vi "main_ctrl.vi"(8 "error in":errorcluster) -> (0 "error out":errorcluster caption="error")   [LabVIEW 2012]
uses:
  <vilib>/Rock Robotics/WPI/DriverStation/WPI_DriverStationRobotMode.ctl
  typedefs/fg_typedef.ctl
  typedefs/vision enable.ctl
  typedefs/subStates.ctl
  typedefs/singleUseSubstate.ctl
  <vilib>/Rock Robotics/WPI/Solenoid/WPI_SolenoidValue.ctl
  <vilib>/Rock Robotics/WPI/Compressor/WPI_CompressorGetSetRefNum.vi
  <vilib>/Rock Robotics/WPI/RobotDrive/WPI_RobotDriveGetSetRefNum.vi
  <vilib>/Rock Robotics/WPI/RobotDrive/WPI_RobotDriveArcadeDrive_Standard(NoSaturation).vi
  <vilib>/Rock Robotics/WPI/Solenoid/WPI_SolenoidSetEnum.vi
panel:
  out "Distance":dbl
  out "Robot Mode":T1
  in  "Output":dbl
  out "Vision SPI":u32
  out "Vision IPS":dbl
  out "Main IPS":dbl
  out "Main SPI":u32
  # "MAIN CONTROL"
  # "holds robot control code - dual parallel state machine"
  # "SPI: milliseconds per iteration\nIPS: iterations per second"
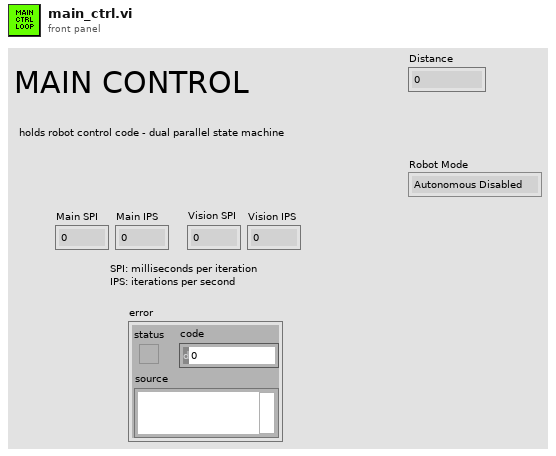
[diagram p1: front panel]
types:
  T1 = typedef "WPI_DriverStationRobotMode.ctl" = enum16{"Autonomous Disabled", "Autonomous Enabled", "Teleop Disabled", "Teleop Enabled", "Timeout", "Finish"}
  T2 = typedef "WPI_SolenoidDevRef.ctl" = cluster{"DevStatus":errorcluster, "Solenoid Module":T3, "Forward Solenoid Channel":T4, "Reverse Solenoid Channel":T4}
  T3 = typedef "FPGA_TypedefSolenoidModule.ctl" = enum16{"Solenoid Module 1", "Solenoid Module 2"}
  T4 = typedef "WPI_SolenoidChannel.ctl" = enum8{"Solenoid 1", "Solenoid 2", "Solenoid 3", "Solenoid 4", "Solenoid 5", "Solenoid 6", "Solenoid 7", "Solenoid 8", "Invalid"}
  T5 = typedef "WPI_CompressorDevRef.ctl" = cluster{"DevStatus":errorcluster, "DigitalInputDevRef":T6, "RelayDevRef":T9}
  T6 = typedef "WPI_DigitalInputDevRef.ctl" = cluster{"DevStatus":errorcluster, "DIO Channel":T7, "Digital Module":T8}
  T7 = typedef "FPGA_DIOChannel.ctl" = enum8{"DIO 1", "DIO 2", "DIO 3", "DIO 4", "DIO 5", "DIO 6", "DIO 7", "DIO 8", "DIO 9", "DIO 10", "DIO 11", "DIO 12", "DIO 13", "DIO 14", "Invalid"}
  T8 = typedef "FPGA_TypedefDigitalModule.ctl" = enum16{"Digital Module 1", "Digital Module 2"}
  T9 = typedef "WPI_RelayDevRef.ctl" = cluster{"DevStatus":errorcluster, "Relay Channel":T10, "Digital Module":T8, "Relay Direction":T11}
  T10 = typedef "FPGA_DIORelayChannel.ctl" = enum8{"Relay 1", "Relay 2", "Relay 3", "Relay 4", "Relay 5", "Relay 6", "Relay 7", "Relay 8", "Invalid"}
  T11 = typedef "WPI_RelayDirection.ctl" = enum16{"Both directions", "Forward only", "Reverse only"}
  T12 = typedef "WPI_MotorControlDeviceRef.ctl" = cluster{"DeviceStatus":errorcluster, "Type":enum16{"PWM", "CAN"}, "PWM":cluster{"Digital Module":T8, "PWM Channel":T13, "DeadBand":T14}, "CAN":cluster{"Device Number":u8, "Control Mode":T15, "Semaphore":T16, "Max Vout":dbl}, "Invert":bool, "TransformRef":T17, "InvTransformRef":T17}
  T13 = typedef "FPGA_DIOPWMChannel.ctl" = enum8{"PWM 1", "PWM 2", "PWM 3", "PWM 4", "PWM 5", "PWM 6", "PWM 7", "PWM 8", "PWM 9", "PWM 10", "Invalid"}
  T14 = typedef "WPI_PWMDeadband.ctl" = cluster{"Name":string, "maxPositivePwm":i32, "minPositivePwm":i32, "centerPwm":i32, "maxNegativePwm":i32, "minNegativePwm":i32, "angularRange":u16}
  T15 = typedef "WPI_CANJaguar_ControlMode.ctl" = enum8{"Percent VBus", "Current", "Speed", "Position", "Voltage"}
  T16 = typedef "Semaphore RefNum" = refnum<k1>
  T17 = typedef "WPI_PWMTransform_ConPane.ctl" = refnum<vi>
  T18 = typedef "WPI_RobotDriveDevRef.ctl" = cluster{"DevStatus":errorcluster, "Motors[]":T12[], "Square Inputs":bool, "Max Output":dbl, "Isochronous":bool}
  T19 = cluster{"Left":dbl, "Top":dbl, "Right":dbl, "Bottom":dbl, "Target CoM X":dbl, "Target CoM Y":dbl}
  T20 = typedef "vision enable.ctl" = enum16{"Enable", "Disable", "Stop"}
  T21 = typedef "fg_typedef.ctl" = enum16{"Get", "Set"}
  T22 = typedef "WPI_CameraDevRef.ctl" = cluster{"Camera Address":string, "CameraStatus":errorcluster, "Acquire Image Notifier":refnum<notifier>}
  T23 = typedef "IMAQ Image.ctl" = refnum<image>
  T24 = cluster{"Vision mSPI":u32, "Main mSPI":u32, "Dash mSPI":u32}
  T25 = typedef "WPI_SolenoidValue.ctl" = enum16{"Off", "On", "Forward", "Reverse"}
  T26 = typedef "singleUseSubstate.ctl" = enum16{"null", "wait", "shift high", "shift low"}
  T27 = typedef "WPI_DriverStationDerivedRobotMode.ctl" = enum16{"Init", "Execute", "Stop"}
  T28 = typedef "subStates.ctl" = enum16{"null", "wait", "driver control", "auto", "manual override", "hold position", "rotate", "feeder", "end"}
  T29 = typedef "Loop 2 Datatype.ctl" = cluster{"State":T28, "Waiting Loop":i32, "State to Wait For":i32, "Loop ID":i32, "Exit Value":i32, "Joystick":dbl}
  T30 = typedef "Loop 1 Datatype.ctl" = cluster{"State":T28, "Waiting Loop":i32, "State to Wait For":i32, "Loop ID":i32, "Exit Value":i32, "Joystick":dbl, "Index Up":bool, "Index Down":bool}
  T31 = typedef "Loop 3 Datatype.ctl" = cluster{"State":T28, "Waiting Loop":i32, "State to Wait For":i32, "Loop ID":i32, "Exit Value":i32, "Joystick":dbl, "Z Axis":dbl}
  T32 = typedef "Loop 0 Datatype.ctl" = cluster{"State":T28, "Waiting Loop":i32, "State to Wait For":i32, "Loop ID":i32, "Exit Value":i32, "X Axis":dbl, "Y Axis":dbl, "Z Axis":dbl}
  T33 = typedef "Loop 4 Datatype.ctl" = cluster{"State":T28, "Waiting Loop":i32, "State to Wait For":i32, "Loop ID":i32, "Exit Value":i32, "Joystick":dbl}
  T34 = typedef "WPI_EncoderDevRef.ctl" = cluster{"DevStatus":errorcluster, "EncoderIndex":T35, "CounterIndex":T36, "DistancePerCount":dbl, "Decoding Type":T37}
  T35 = typedef "FPGA_EncoderIdx.ctl" = enum8{"Enc 0", "Enc 1", "Enc 2", "Enc 3", "Invalid"}
  T36 = typedef "FPGA_CounterCtrSystemIndex.ctl" = enum8{"Ctr 0", "Ctr 1", "Ctr 2", "Ctr 3", "Ctr 4", "Ctr 5", "Ctr 6", "Ctr 7", "Invalid"}
  T37 = typedef "WPI_EncoderType.ctl" = enum16{"1x", "2x", "4x"}
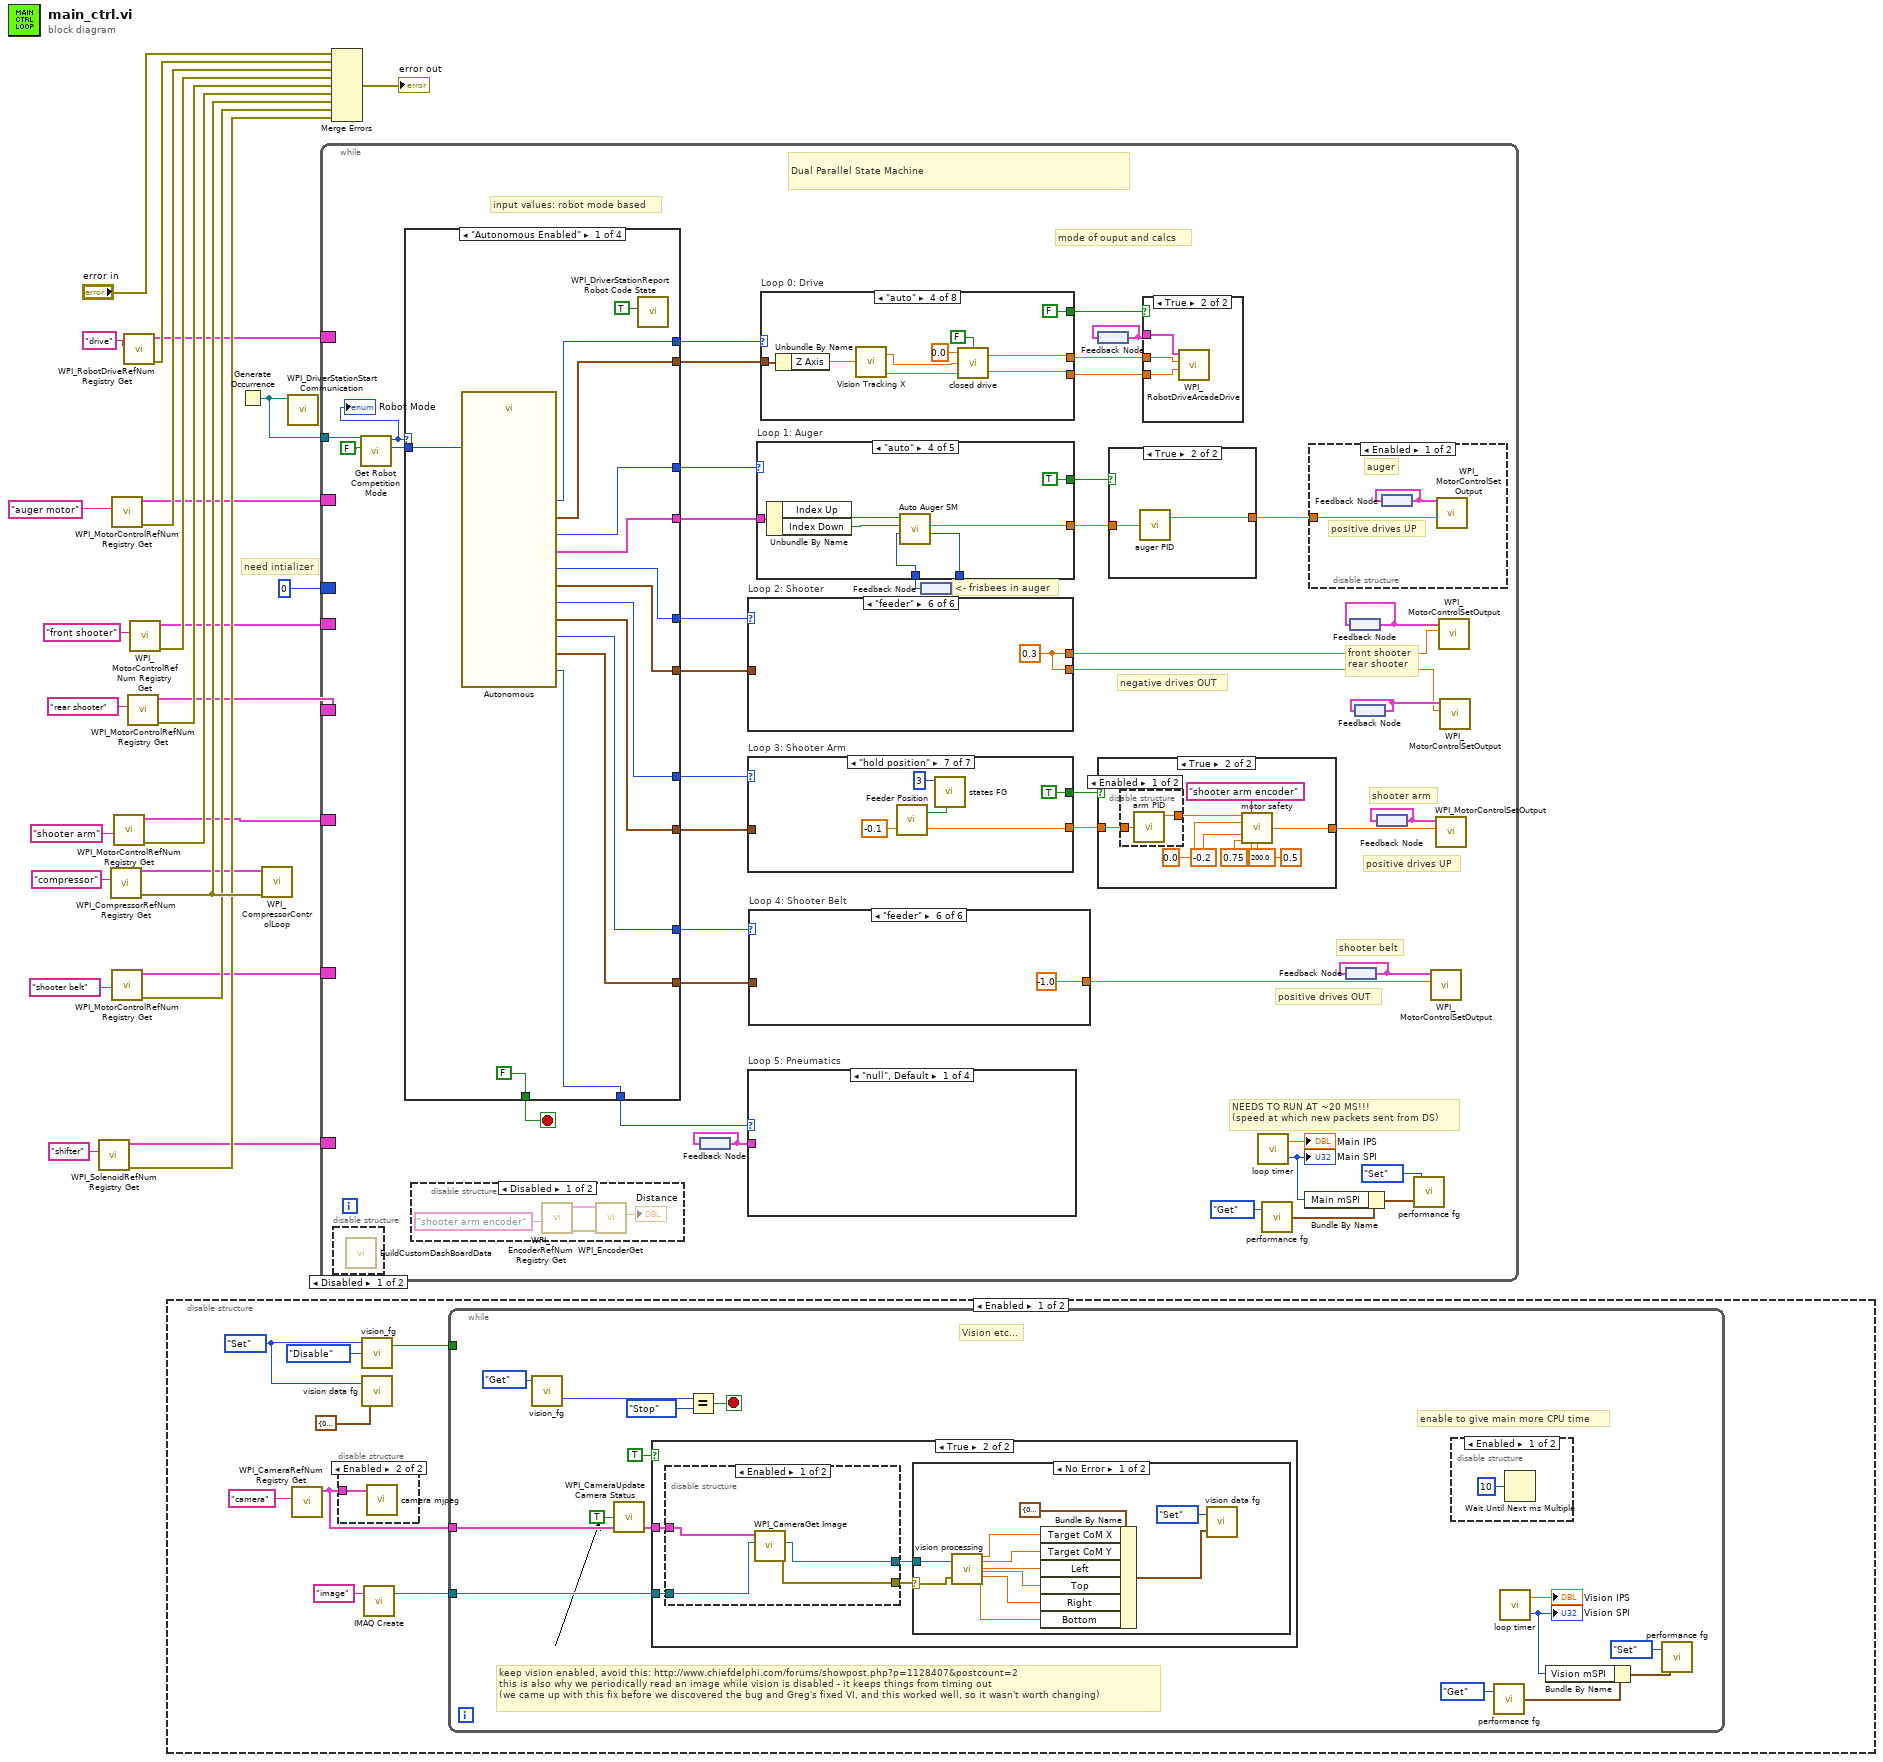
[diagram p0: block diagram]
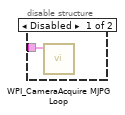
[diagram p2: hidden frame]
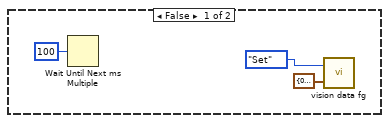
[diagram p4: hidden frame]
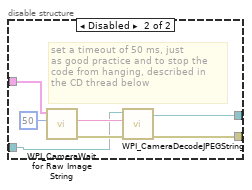
[diagram p6: hidden frame]
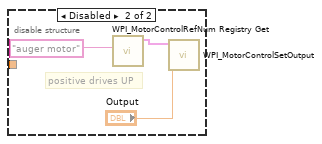
[diagram p10: hidden frame]
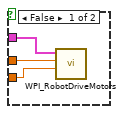
[diagram p13: hidden frame]
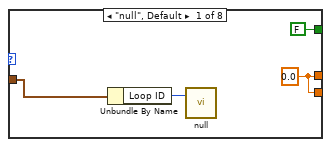
[diagram p14: hidden frame]
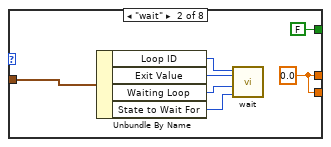
[diagram p15: hidden frame]
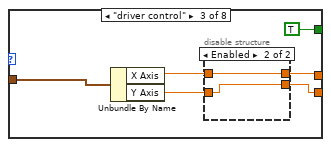
[diagram p16: hidden frame]
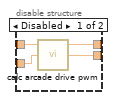
[diagram p17: hidden frame]
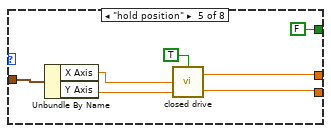
[diagram p18: hidden frame]
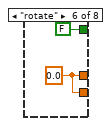
[diagram p19: hidden frame]
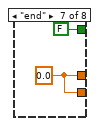
[diagram p20: hidden frame]
diagram:
  # "need intializer"
  n1 = call <vilib>:"WPI_SolenoidRefNum Registry Get.vi"("refnum name"="shifter") -> ("error out"=w12:errorcluster, "SolenoidDevRef"=w4:T2)  [unwired: 9 in]
  n2 = call <vilib>:"WPI_CompressorRefNum Registry Get.vi"("refnum name"="compressor") -> ("error out"=w14:errorcluster, "CompressorDevRef"=w6:T5)  [unwired: 9 in]
  n3 = call <vilib>:"WPI_MotorControlRefNum Registry Get.vi"("refnum name"="auger motor") -> ("error out"=w18:errorcluster, "MotorControlDevRef"=w10:T12)  [unwired: 9 in]
  n4 = call <vilib>:"WPI_MotorControlRefNum Registry Get.vi"("refnum name"="shooter belt") -> ("error out"=w13:errorcluster, "MotorControlDevRef"=w5:T12)  [unwired: 9 in]
  n5 = call <vilib>:"WPI_MotorControlRefNum Registry Get.vi"("refnum name"="shooter arm") -> ("error out"=w15:errorcluster, "MotorControlDevRef"=w7:T12)  [unwired: 9 in]
  n6 = call <vilib>:"WPI_RobotDriveRefNum Registry Get.vi"("refnum name"="drive") -> ("error out"=w20:errorcluster, "RobotDriveDevRef"=w11:T18)  [unwired: 9 in]
  n7 = call <vilib>:"WPI_MotorControlRefNum Registry Get.vi"("refnum name"="rear shooter") -> ("error out"=w16:errorcluster, "MotorControlDevRef"=w8:T12)  [unwired: 9 in]
  n8 = call <vilib>:"WPI_MotorControlRefNum Registry Get.vi"("refnum name"="front shooter") -> ("error out"=w17:errorcluster, "MotorControlDevRef"=w9:T12)  [unwired: 9 in]
  n9 = disable-structure shown="Enabled" {
    frame Enabled {
      w34 = fg_typedef."Set" ("Enum")
      n10 = call <vilib>:"WPI_CameraRefNum Registry Get.vi"("refnum name"="camera") -> ("CameraDevRef"=w31:T22)  [unwired: 9 in, 1 out]
      n11 = disable-structure shown="Enabled" {
        disable-tunnel: w31 -> [w37 w38]
        frame Disabled {
          n12 = call <vilib>:"WPI_CameraAcquire MJPG Loop.vi"("CameraDevRef"=w37) -> ()  [unwired: 11 in]
        }
        frame Enabled {
          n13 = call "camera mjpeg.vi"("CameraDevRef"=w38) -> ()  [unwired: 11 in]
        }
      }
      n14 = call "vision_fg.vi"("Action"=vision_enable."Disable", "Menu"=w34) -> ("Enabled?"=w35:bool)  [unwired: 1 in, 1 out]
      n15 = call "vision data fg.vi"("Input"=T19 {"Left"=0.0, "Top"=0.0, "Right"=0.0, "Bottom"=0.0, "Target CoM X"=0.0, "Target CoM Y"=0.0}, "Menu"=w34) -> ()  [unwired: 1 out]
      n16 = call "IMAQ Create"("Image Name"="image") -> ("New Image"=w36:T23)  [unwired: 4 in, 1 out]
      n17 = while {
        tunnel: w36 -> [w52]
        tunnel: w31 -> [w51]
        tunnel: w35 -> [_]
        stop <- w53 stop-if-true
        # "keep vision enabled, avoid this: http://www.chiefdelphi.com/forums/showpost.php?p=1128407&postcount=2\nthis is also why we periodically read an image while vision is disabled - it keeps things from timing out\n(we came up with this fix before we discovered the bug and Greg's fixed VI, and this worked well, so it wasn't worth changing)"
        # "enable to give main more CPU time"
        # "Vision etc..."
        n18 = call "vision_fg.vi"("Menu"=fg_typedef."Get" ("Enum")) -> ("State Out"=w47:T20)  [unwired: 2 in, 1 out]
        n19 = call <vilib>:"WPI_CameraUpdate Camera Status.vi"("CameraDevRef In"=w51, "Enable Vision"=TRUE) -> ("CameraDevRef Out"=w50:T22)  [unwired: 3 in]
        n20 = case shown="True" TRUE {
          tunnel: w52 -> [_ w61]
          tunnel: w50 -> [_ w60]
          frame False {
            n21 = Wait Until Next ms Multiple(millisecond multiple=u32 100) -> ()  [unwired: 1 out]
            n22 = call "vision data fg.vi"("Input"=T19 {"Left"=0.0, "Top"=0.0, "Right"=0.0, "Bottom"=0.0, "Target CoM X"=0.0, "Target CoM Y"=0.0}, "Menu"=fg_typedef."Set" ("Enum")) -> ()  [unwired: 1 out]
          }
          frame True {
            n23 = disable-structure shown="Enabled" {
              disable-tunnel: w61 -> [w75 w79]
              disable-tunnel: w60 -> [w76 w81]
              disable-tunnel: [w74 w78] -> w59
              disable-tunnel: [w73 w77] -> w58
              frame Enabled {
                n24 = call <vilib>:"WPI_CameraGet Image.vi"("Image"=w75, "CameraDevRef"=w76) -> ("error out"=w73:errorcluster, "Image Out"=w74:T23)  [unwired: 7 in, 1 out]
              }
              frame Disabled {
                # "set a timeout of 50 ms, just\nas good practice and to stop the \ncode from hanging, described in \nthe CD thread below"
                n25 = call <vilib>:"WPI_CameraWait for Raw Image String.vi"("Timeout in ms (-1)"=50, "CameraDevRef"=w81) -> ("error out"=w83:errorcluster, "String"=w82:string)  [unwired: 3 in, 5 out]
                n26 = call <vilib>:"WPI_CameraDecodeJPEGString.vi"("error in"=w83, "Compressed Image"=w82, "Image In"=w79) -> ("error out"=w77:errorcluster, "Image Out"=w78:T23)  [unwired: 3 out]
              }
            }
            n27 = case shown="No Error" w58 {
              selector: w58 -> [w70 _]
              tunnel: w59 -> [w71 _]
              frame No Error {
                n28 = call "vision processing.vi"("Image In"=w71, "error in (no error)"=w70) -> ("x"=w69:dbl, "y"=w68:dbl, "left"=w66:dbl, "top"=w65:dbl, "right"=w64:dbl, "bottom"=w63:dbl)  [unwired: 11 in, 1 out]
                n29 = Bundle By Name(cluster=T19 {"Left"=0.0, "Top"=0.0, "Right"=0.0, "Bottom"=0.0, "Target CoM X"=0.0, "Target CoM Y"=0.0} ("Input"), "Target CoM X"=w69, "Target CoM Y"=w68, "Left"=w66, "Top"=w65, "Right"=w64, "Bottom"=w63) -> (w62:T19)
                n30 = call "vision data fg.vi"("Input"=w62, "Menu"=fg_typedef."Set" ("Enum")) -> ()  [unwired: 1 out]
              }
              frame Error {
              }
            }
          }
        }
        n31 = Equal?(x=w47, y=vision_enable."Stop") -> (x = y?=w53:bool)
        n32 = disable-structure shown="Enabled" {
          frame Enabled {
            n33 = Wait Until Next ms Multiple(millisecond multiple=u32 10) -> ()  [unwired: 1 out]
          }
          frame Disabled {
          }
        }
        n34 = call "performance fg.vi"("Menu"=fg_typedef."Get") -> ("Output"=w43:T24)  [unwired: 1 in]
        n35 = call "loop timer.vi"() -> ("IPS"=→"Vision IPS":dbl, "SPI"=w45:u32)  [unwired: 1 in]
        "Vision SPI" <- w45
        n36 = Bundle By Name(cluster=w43, "Vision mSPI"=w45) -> (w42:T24)
        n37 = call "performance fg.vi"("Input"=w42, "Menu"=fg_typedef."Set") -> ()  [unwired: 1 out]
      }
    }
    frame Disabled {
    }
  }
  n38 = Generate Occurrence() -> (w28:refnum<k4>)
  n39 = call <vilib>:"WPI_CompressorControlLoop.vi"("error in (no error)"=w14, "CompressorDevRef"=w6) -> ()  [unwired: 10 in]
  n40 = call <vilib>:"WPI_DriverStationStart Communication.vi"("occurrence"=w28) -> ()  [unwired: 11 out]
  n41 = while {
    tunnel: w28 -> [w124]
    border: w8 -> [_]
    border: w9 -> [_]
    border: w10 -> [_]
    border: w11 -> [_]
    border: w4 -> [_]
    border: w5 -> [_]
    border: w7 -> [_]
    border: i8 0 -> [_]
    stop <- w118 stop-if-true
    # "positive drives UP"
    # "shooter arm"
    # "<- frisbees in auger"
    # "positive drives OUT"
    # "negative drives OUT"
    # "front shooter\nrear shooter"
    # "shooter belt"
    # "input values: robot mode based"
    # "mode of ouput and calcs"
    # "NEEDS TO RUN AT ~20 MS!!!\n(speed at which new packets sent from DS)"
    # "Dual Parallel State Machine"
    n42 = disable-structure shown="Disabled" {
      frame Disabled {
        n43 = call "BuildCustomDashBoardData.vi"() -> ()  [unwired: 12 in]
      }
      frame Enabled {
      }
    }
    n44 = call "Get Robot Competition Mode.vi"("Finish"=FALSE, "DS Occurrence"=w124) -> ("Call Context"=w122:T27, "Robot Mode"=w123:T1)  [unwired: 6 in, 2 out]
    "Robot Mode" <- w123
    n45 = case shown="\"Autonomous Enabled\"" w123 {
      tunnel: [w327 w345 w346 w352] -> w87
      tunnel: w122 -> [w318 w340 _ _]
      tunnel: [w325 w344 w346 w352] -> w120
      tunnel: [w319 w342 singleUseSubstate."null" ("SubState 5") singleUseSubstate."null" ("SubState 5")] -> w119
      tunnel: [FALSE FALSE FALSE TRUE] -> w118
      tunnel: [w329 w339 w346 w352] -> w111
      tunnel: [w328 w338 _ _] -> w112
      tunnel: [w326 w337 _ _] -> w110
      tunnel: [w324 w336 _ _] -> w109
      tunnel: [w322 w335 _ _] -> w102
      tunnel: [w320 w334 _ _] -> w101
      tunnel: [w321 w333 w346 w352] -> w100
      tunnel: [w323 w332 w346 w352] -> w99
      frame "Autonomous Enabled" {
        n46 = call "Autonomous.vi"("Call Context"=w318) -> ("SubState 2"=w325:T28, "Loop 2 Data"=w324:T29, "SubState 1"=w327:T28, "Loop 1 Data"=w326:T30, "Loop 3 Data"=w322:T31, "SubState 0"=w329:T28, "SubState 3"=w323:T28, "Loop 0 Data"=w328:T32, "Loop 4 Data"=w320:T33, "SubState 4"=w321:T28, "SubState 5"=w319:T26)
        n47 = call <vilib>:"WPI_DriverStationReport Robot Code State.vi"("Autonomous"=TRUE) -> ()  [unwired: 10 in, 1 out]
      }
      frame "Teleop Enabled" {
        n48 = call "Teleop.vi"("Call Context"=w340) -> ("SubState 3"=w332:T28, "SubState 4"=w333:T28, "SubState 5"=w342:T26, "Loop 3 Data"=w335:T31, "Loop 4 Data"=w334:T33, "SubState 0"=w339:T28, "Loop 1 Data"=w337:T30, "Loop 0 Data"=w338:T32, "SubState 1"=w345:T28, "Loop 2 Data"=w336:T29, "SubState 2"=w344:T28)  [unwired: 8 in]
        n49 = call <vilib>:"WPI_DriverStationReport Robot Code State.vi"("TeleOp"=TRUE) -> ()  [unwired: 10 in, 1 out]
      }
      frame "Autonomous Disabled", "Teleop Disabled", "Timeout" {
        w346 = subStates."null" ("SubState 0")
        # "set all loops to null"
        # "make sure to disable vision\nwe don't need it here"
        # "robot disabled, timeout"
        n50 = call "vision_fg.vi"("Action"=vision_enable."Disable", "Menu"=fg_typedef."Set") -> ()  [unwired: 1 in, 2 out]
        n51 = call <vilib>:"WPI_DriverStationReport Robot Code State.vi"("Disabled"=TRUE) -> ()  [unwired: 10 in, 1 out]
      }
      frame "Finish" {
        w352 = subStates."end"  # Stop All Loops
        # "stop the while loop"
        # "stop DS comms"
        # "stop vision loop"
        n52 = call <vilib>:"WPI_DriverStationStop Communication.vi"("StopCommunication"=TRUE) -> ()  [unwired: 10 in, 1 out]
        n53 = call "vision_fg.vi"("Action"=vision_enable."Stop", "Menu"=fg_typedef."Set") -> ()  [unwired: 1 in, 2 out]
      }
    }
    n54 = disable-structure shown="Disabled" {
      frame Disabled {
        n55 = call <vilib>:"WPI_EncoderRefNum Registry Get.vi"("refnum name"="shooter arm encoder") -> ("error out"=w128:errorcluster, "EncoderDevRef"=w127:T34)  [unwired: 9 in]
        n56 = call <vilib>:"WPI_EncoderGet.vi"("error in (no error)"=w128, "EncoderDevRef"=w127) -> ("Distance"=→"Distance":dbl)  [unwired: 4 in, 5 out]
      }
      frame Enabled {
      }
    }
    n57 = feedback #1() -> (w104:T2)
    n58 = feedback-in #1(w104) -> ()
    n59 = case "Loop 2: Shooter" shown="\"feeder\"" w120 {
      tunnel: w109 -> [w273 w275 _ w282 _ _]
      tunnel: [w271 w274 w280 w281 -1.0 ("Joystick") w285] -> w105
      tunnel: [w271 w274 w280 w281 -0.8 ("Joystick") w285] -> w89
      frame "null", Default {
        w271 = 0.0 ("Joystick")
        n60 = Unbundle By Name(w273) -> ("Loop ID"=w272:i32)
        n61 = call "null.vi"("This Loop ID"=w272) -> ()  [unwired: 2 in]
      }
      frame "wait" {
        w274 = 0.0 ("Joystick")
        n62 = Unbundle By Name(w275) -> ("Loop ID"=w279:i32, "Exit Value"=w278:i32, "Waiting Loop"=w277:i32, "State to Wait For"=w276:i32)
        n63 = call "wait.vi"("State to wait for"=w276, "Waiting Loop ID"=w277, "time (ms)"=w278, "Current Loop ID"=w279) -> ()  [unwired: 1 out]
      }
      frame "driver control" {
        w280 = 0.0
      }
      frame "manual override" {
        n64 = Unbundle By Name(w282) -> ("Joystick"=w281:dbl)
      }
      frame "auto" {
      }
      frame "feeder" {
        w285 = 0.3 ("Joystick")
      }
    }
    n65 = case "Loop 3: Shooter Arm" shown="\"hold position\"" w99 {
      tunnel: w102 -> [w222 w225 w233 w240 w243 w255 _]
      tunnel: [0.0 ("Joystick") 0.0 ("Joystick") w231 w238 w244 w257 w263] -> w92
      tunnel: [FALSE FALSE TRUE FALSE TRUE TRUE ("Boolean") TRUE ("Boolean")] -> w90
      frame "null", Default {
        n66 = Unbundle By Name(w222) -> ("Loop ID"=w221:i32)
        n67 = call "null.vi"("This Loop ID"=w221) -> ()  [unwired: 2 in]
      }
      frame "wait" {
        n68 = Unbundle By Name(w225) -> ("Loop ID"=w229:i32, "Exit Value"=w228:i32, "Waiting Loop"=w227:i32, "State to Wait For"=w226:i32)
        n69 = call "wait.vi"("State to wait for"=w226, "Waiting Loop ID"=w227, "time (ms)"=w228, "Current Loop ID"=w229) -> ()  [unwired: 1 out]
      }
      frame "driver control" {
        n70 = Unbundle By Name(w233) -> ("Joystick"=w230:dbl)
        n71 = disable-structure shown="Enabled" {
          disable-tunnel: w230 -> [w235 w236]
          disable-tunnel: [w234 w236] -> w231
          frame Enabled {
            n72 = call "arm hold.vi"("Input"=w235) -> ("Rate Out"=w234:dbl)
          }
          frame Disabled {
          }
        }
      }
      frame "manual override" {
        n73 = Unbundle By Name(w240) -> ("Joystick"=w239:dbl)
        n74 = expression code="x/2"(w239) -> (w238:dbl)
      }
      frame "auto" {
        n75 = Unbundle By Name(w243) -> ("Z Axis"=w242:dbl)
        n76 = local read "Robot Mode"() -> (w241:T1)
        n77 = disable-structure shown="Enabled" {
          disable-tunnel: [w252 w253] -> w245
          disable-tunnel: w242 -> [w251 w253]
          disable-tunnel: w241 -> [w250 _]
          frame Enabled {
            n78 = call "VisionTracking Y.vi"("Robot Mode"=w250, "Tweak"=w251) -> ("output"=w252:dbl)
          }
          frame Disabled {
          }
        }
        n79 = disable-structure shown="Enabled" {
          disable-tunnel: w245 -> [w248 w249]
          disable-tunnel: [w247 w249] -> w244
          frame Disabled {
            n80 = call "arm hold.vi"("Input"=w248) -> ("Rate Out"=w247:dbl)
          }
          frame Enabled {
          }
        }
      }
      frame "feeder" {
        n81 = Unbundle By Name(w255) -> ("Z Axis"=w254:dbl)
        n82 = call "Feeder Position.vi"("setpoint"=-0.135, "Z Axis"=w254) -> ("Rate"=w257:dbl)  [unwired: 1 out]
      }
      frame "hold position" {
        n83 = call "Feeder Position.vi"("setpoint"=-0.1) -> ("Rate"=w263:dbl, "Finished"=w260:bool)  [unwired: 1 in]
        n84 = call "states FG.vi"("exit in"=w260, "Loop ID"=3) -> ()  [unwired: 6 in, 4 out]
      }
    }
    n85 = case "Loop 5: Pneumatics" shown="\"null\", Default" w119 {
      tunnel: w104 -> [_ _ w268 w269]
      frame "null", Default {
      }
      frame "wait" {
      }
      frame "shift high" {
        n86 = call-poly <vilib>:"WPI_SolenoidSet.vi"("Value"=WPI_SolenoidValue."Forward", "SolenoidDevRef"=w268) -> ()  [unwired: 8 in, 2 out]
      }
      frame "shift low" {
        n87 = call-poly <vilib>:"WPI_SolenoidSet.vi"("Value"=WPI_SolenoidValue."Reverse", "SolenoidDevRef"=w269) -> ()  [unwired: 8 in, 2 out]
      }
    }
    n88 = case "Loop 4: Shooter Belt" shown="\"feeder\"" w100 {
      tunnel: w101 -> [w205 w207 w213 w216 _ _]
      tunnel: [0.0 ("Joystick") 0.0 ("Joystick") w212 w214 1.0 ("Joystick") -1.0 ("Joystick")] -> w103
      frame "null", Default {
        n89 = Unbundle By Name(w205) -> ("Loop ID"=w204:i32)
        n90 = call "null.vi"("This Loop ID"=w204) -> ()  [unwired: 2 in]
      }
      frame "wait" {
        n91 = Unbundle By Name(w207) -> ("Loop ID"=w211:i32, "Exit Value"=w210:i32, "Waiting Loop"=w209:i32, "State to Wait For"=w208:i32)
        n92 = call "wait.vi"("State to wait for"=w208, "Waiting Loop ID"=w209, "time (ms)"=w210, "Current Loop ID"=w211) -> ()  [unwired: 1 out]
      }
      frame "driver control" {
        n93 = Unbundle By Name(w213) -> ("Joystick"=w212:dbl)
      }
      frame "manual override" {
        n94 = Unbundle By Name(w216) -> ("Joystick"=w215:dbl)
        n95 = expression code="x/2"(w215) -> (w214:dbl)
      }
      frame "auto" {
      }
      frame "feeder" {
      }
    }
    n96 = case "Loop 0: Drive" shown="\"auto\"" w111 {
      tunnel: w112 -> [w156 w160 w170 w178 w191 _ _ w202]
      tunnel: [w154 w158 w166 w184 w188 w194 w196 w198] -> w96
      tunnel: [w154 w158 w165 w183 w187 w194 w196 w197] -> w95
      tunnel: [FALSE FALSE TRUE FALSE FALSE FALSE FALSE FALSE] -> w97
      frame "null", Default {
        w154 = 0.0 ("X Axis")
        n97 = Unbundle By Name(w156) -> ("Loop ID"=w157:i32)
        n98 = call "null.vi"("This Loop ID"=w157) -> ()  [unwired: 2 in]
      }
      frame "wait" {
        w158 = 0.0 ("X Axis")
        n99 = Unbundle By Name(w160) -> ("Loop ID"=w164:i32, "Exit Value"=w163:i32, "Waiting Loop"=w162:i32, "State to Wait For"=w161:i32)
        n100 = call "wait.vi"("State to wait for"=w161, "Waiting Loop ID"=w162, "time (ms)"=w163, "Current Loop ID"=w164) -> ()  [unwired: 1 out]
      }
      frame "driver control" {
        n101 = Unbundle By Name(w170) -> ("X Axis"=w168:dbl, "Y Axis"=w167:dbl)
        n102 = disable-structure shown="Enabled" {
          disable-tunnel: w168 -> [w174 w176]
          disable-tunnel: w167 -> [w173 w175]
          disable-tunnel: [w172 w176] -> w166
          disable-tunnel: [w171 w175] -> w165
          frame Disabled {
            n103 = call "calc arcade drive pwm.vi"("Y axis value"=w173, "X axis value"=w174) -> ("Right Speed"=w171:dbl, "Left Speed"=w172:dbl)  [unwired: 1 in, 1 out]
          }
          frame Enabled {
          }
        }
      }
      frame "auto" {
        n104 = Unbundle By Name(w178) -> ("Z Axis"=w177:dbl)
        n105 = call "Vision Tracking X.vi"("Tweak"=w177) -> ("right speed"=w181:dbl, "left speed"=w180:dbl)
        n106 = call "closed drive.vi"("Acrade Drive?"=FALSE, "Y axis value (Left)"=w180, "X axis value (Right)"=w181, "Threshold (.4)"=0.0 ("Threshold")) -> ("right"=w183:dbl, "left"=w184:dbl)
      }
      frame "hold position" {
        n107 = Unbundle By Name(w191) -> ("X Axis"=w190:dbl, "Y Axis"=w189:dbl)
        n108 = call "closed drive.vi"("Acrade Drive?"=TRUE, "Y axis value (Left)"=w189, "X axis value (Right)"=w190) -> ("right"=w187:dbl, "left"=w188:dbl)  [unwired: 1 in]
      }
      frame "rotate" {
        w194 = 0.0 ("X Axis")
      }
      frame "end" {
        w196 = 0.0 ("X Axis")
      }
      frame "manual override" {
        n109 = Unbundle By Name(w202) -> ("X Axis"=w201:dbl, "Y Axis"=w200:dbl)
        n110 = expression code="x/2"(w201) -> (w198:dbl)
        n111 = expression code="x/2"(w200) -> (w197:dbl)
      }
    }
    n112 = feedback #2() -> (w88:i8)
    n113 = case "Loop 1: Auger" shown="\"auto\"" w87 {
      tunnel: w110 -> [w288 w293 w303 w311 w316]
      tunnel: [0.0 ("Y Axis") 0.0 ("Y Axis") w304 w312 w314] -> w108
      tunnel: [FALSE FALSE TRUE TRUE FALSE] -> w107
      tunnel: w88 -> [w286 w291 w301 w310 w313]
      tunnel: [w286 w291 w300 w309 w313] -> w85
      frame "null", Default {
        n114 = Unbundle By Name(w288) -> ("Loop ID"=w290:i32)
        n115 = call "null.vi"("This Loop ID"=w290) -> ()  [unwired: 2 in]
      }
      frame "wait" {
        n116 = Unbundle By Name(w293) -> ("Loop ID"=w298:i32, "Exit Value"=w297:i32, "Waiting Loop"=w296:i32, "State to Wait For"=w295:i32)
        n117 = call "wait.vi"("State to wait for"=w295, "Waiting Loop ID"=w296, "time (ms)"=w297, "Current Loop ID"=w298) -> ()  [unwired: 1 out]
      }
      frame "driver control" {
        n118 = Unbundle By Name(w303) -> ("Index Up"=w299:bool, "Index Down"=w302:bool)
        n119 = call "auto auger.vi"("Number of Frisbees"=w301, "Index Down"=w302, "Index Up"=w299) -> ("Number of Frisbees Out"=w300:i8, "Setpoint Out"=w304:dbl)  [unwired: 1 out]
      }
      frame "auto" {
        n120 = Unbundle By Name(w311) -> ("Index Up"=w307:bool, "Index Down"=w308:bool)
        n121 = call "Auto Auger SM.vi"("Frisbees In"=w310, "Index Down"=w308, "Index Up"=w307) -> ("Number of Frisbees Out"=w309:i8, "Setpoint Out"=w312:dbl)  [unwired: 7 in]
      }
      frame "manual override" {
        n122 = Unbundle By Name(w316) -> ("Joystick"=w315:dbl)
        n123 = expression code="x/2"(w315) -> (w314:dbl)
      }
    }
    n124 = feedback-in #2(w85) -> ()
    n125 = feedback #3() -> (w94:T18)
    n126 = feedback-in #3(w94) -> ()
    n127 = case shown="True" w90 {
      tunnel: w92 -> [w135 w144]
      tunnel: [w135 w140] -> w91
      frame False {
      }
      frame True {
        n128 = disable-structure shown="Enabled" {
          disable-tunnel: w144 -> [w146 w147]
          disable-tunnel: [w145 w147] -> w143
          frame Enabled {
            n129 = call "arm PID.vi"("Desired Rate"=w146) -> ("Motor Output"=w145:dbl)  [unwired: 3 in]
          }
          frame Disabled {
          }
        }
        n130 = call "motor safety.vi"("Desired Rate"=w143, "Encoder Refnum"="shooter arm encoder" ("refnum name"), "Forward Limit"=0.0, "Reverse Limit"=-0.2, "Cutoff Rate"=0.75, "Max Rate"=200.0, "Min Rate"=0.5) -> ("Rate Output"=w140:dbl)  [unwired: 8 in]
      }
    }
    n131 = case shown="True" w107 {
      tunnel: w108 -> [w264 w266]
      tunnel: [w264 w265] -> w106
      frame False {
      }
      frame True {
        n132 = call "auger PID.vi"("setpoint"=w266) -> ("output"=w265:dbl)  [unwired: 1 in]
      }
    }
    n133 = case shown="True" w97 {
      tunnel: w96 -> [w149 w153]
      tunnel: w95 -> [w148 w152]
      tunnel: w94 -> [w150 w151]
      frame False {
        n134 = call <vilib>:"WPI_RobotDriveMotors.vi"("RightSpeed"=w148, "LeftSpeed"=w149, "RobotDriveDevRef"=w150) -> ()  [unwired: 6 in, 3 out]
      }
      frame True {
        n135 = call-poly <vilib>:"WPI_RobotDriveArcadeDrive.vi"("Y axis value"=w152, "X axis value"=w153, "RobotDriveDevRef"=w151) -> ()  [unwired: 6 in, 3 out]
      }
    }
    n136 = call "loop timer.vi"() -> ("IPS"=→"Main IPS":dbl, "SPI"=w117:u32)  [unwired: 1 in]
    "Main SPI" <- w117
    n137 = call "performance fg.vi"("Menu"=fg_typedef."Get") -> ("Output"=w114:T24)  [unwired: 1 in]
    n138 = Bundle By Name(cluster=w114, "Main mSPI"=w117) -> (w113:T24)
    n139 = disable-structure shown="Enabled" {
      disable-tunnel: w106 -> [w131 _]
      frame Enabled {
        # "positive drives UP"
        # "auger"
        n140 = feedback #4() -> (w130:T12)
        n141 = feedback-in #4(w130) -> ()
        n142 = call <vilib>:"WPI_MotorControlSetOutput.vi"("Output"=w131, "MotorControlDevRef"=w130) -> ()  [unwired: 7 in, 3 out]
      }
      frame Disabled {
        # "positive drives UP"
        n143 = call <vilib>:"WPI_MotorControlRefNum Registry Get.vi"("refnum name"="auger motor") -> ("MotorControlDevRef"=w133:T12)  [unwired: 9 in, 1 out]
        n144 = call <vilib>:"WPI_MotorControlSetOutput.vi"("Output"="Output", "MotorControlDevRef"=w133) -> ()  [unwired: 7 in, 3 out]
      }
    }
    n145 = feedback #5() -> (w84:T12)
    n146 = feedback-in #5(w84) -> ()
    n147 = feedback #6() -> (w93:T12)
    n148 = feedback-in #6(w93) -> ()
    n149 = feedback #7() -> (w98:T12)
    n150 = feedback-in #7(w98) -> ()
    n151 = feedback #8() -> (w86:T12)
    n152 = feedback-in #8(w86) -> ()
    n153 = call "performance fg.vi"("Input"=w113, "Menu"=fg_typedef."Set") -> ()  [unwired: 1 out]
    n154 = call <vilib>:"WPI_MotorControlSetOutput.vi"("Output"=w103, "MotorControlDevRef"=w84) -> ()  [unwired: 7 in, 3 out]
    n155 = call <vilib>:"WPI_MotorControlSetOutput.vi"("Output"=w91, "MotorControlDevRef"=w86) -> ()  [unwired: 7 in, 3 out]
    n156 = call <vilib>:"WPI_MotorControlSetOutput.vi"("Output"=w105, "MotorControlDevRef"=w93) -> ()  [unwired: 7 in, 3 out]
    n157 = call <vilib>:"WPI_MotorControlSetOutput.vi"("Output"=w89, "MotorControlDevRef"=w98) -> ()  [unwired: 7 in, 3 out]
  }
  n158 = Merge Errors("error in", w20, w18, w17, w16, w15, w14, w13, w12) -> (→"error out":errorcluster)
